vi "OPO Monitor.vi"() -> ()   [LabVIEW 2009]
doc: "Example: Simulated Acquisition\n\nRecommended Input Signal: None\n\nDevices Supported: NI 5102, NI 5911, NI 5112, NI 5620, NI 5621, NI 5122, NI 5124, NI 5922, NI 5114, NI 5142 (562x devices require configuration of a 2 V vertical range, 50 ohm input impedance and appropriate vertical coupling).\n\nDescription:\n\nThis example simulates an acquisition on the selected digitizer. To select a digitizer choose a model and a board type from the menu rings. Not all models support all board types. For example, there is only a PXI-5620, but there all the board types exist for a NI-5102.\n\nThis example configures all the digitizer's vertical, horizontal, and triggering properties before every acquisition. It allows you to experiment with numerous configurations, including some triggering modes, since it supports nearly the entire functionality of NI-SCOPE.\n\nMany parameters are included an the front panel of this example. Notice that the \"min sample rate\" is next to the \"actual sample rate,\" and similarly the \"min record length\" is near the \"actual record length.\" The \"min\" values are specified with the Configure Horizontal Timing VI. NI-SCOPE maintains a constant time per record for each acquisition. So when you specify a min sample rate and a min record length, this determines the amount of time the acquisition should take:\n\n time per record = min record length / min sampling rate. \n\nHowever, digitizers support only a certain number of defined sampling rates, so if the value chosen is not a valid rate, it is rounded to the next higher rate, called the actual sample rate. The actual record length is then calculated in order to maintain the time per record. Both of these values are returned in this example so you can investigate the effects of parameter rounding with your digitizer. For more information about parameter coercions, see the NI High Speed Digitizers Help.\n\nThe enforce realtime property allows this example to use Random Interleaved Sampling. See the Random Interleaved Sampling example for more details.\n\nKeep in mind that not all digitizers support all the features in this example. The NI High Speed Digitizers Help includes a table of supported features for each device."
uses:
  <instrlib>/niScope/Controls/niScope vertical coupling.ctl
  Pulse Acquisition/5122-States.ctl
  <instrlib>/niScope/Configure/Trigger/niScope Configure Trigger Edge.vi
  <instrlib>/niScope/Acquire/Fetch/niScope Fetch.vi
  <vilib>/Utility/file.llb/Write To Spreadsheet File (DBL).vi
panel:
  in  "Resource name 5":refnum<k15>="Dev2" caption="Resource Name"
  in  "Channel name (0 or 1) 6":string="0" caption="Channel Name(s)"
  in  "Vertical range (0 to 10V) 6":dbl=0.2 caption="Vertical Range (V)" format="%.2f"
  in  "Sample rate 6":dbl=100000000.0 caption="Min. Sample Rate" step=1000000.0 format="%.3p"
  in  "Number of points\n(max 23500000 si \n100 Ms/s) 5":i32=1000000 caption="Min. Record Length"
  in  "Trigger slope 6":i32(ring) caption="Trigger Slope" items=["Positive", "Negative"]
  in  "Trigger level 5":dbl=0.5 caption="Trigger Level" format="%.2f"
  in  "Trigger source 5":string(combo)="VAL_EXTERNAL" caption="Trigger Source"
  in  "Vertical coupling 6":T1 caption="Vertical Coupling" items=["AC", "DC", "Ground"]
  out "Acquisition time (s) 5":dbl
  in  "Delay trig to acquisition (s) 5":dbl=0.0001 format="%#_7e"
  in  "Capture":bool
  in  "Stop acquisition":bool
  in  "File where data is written":path=path "C:/Users/atomes/Documents/Manips/Labview manip/SQZ/Acquisition brute carte/Data acquisition.txt"
  out "Acquisition brute carte":dbl[](graph)
  # "General"
  # "Timing control"
  # "Trigger"
  # "Vertical"
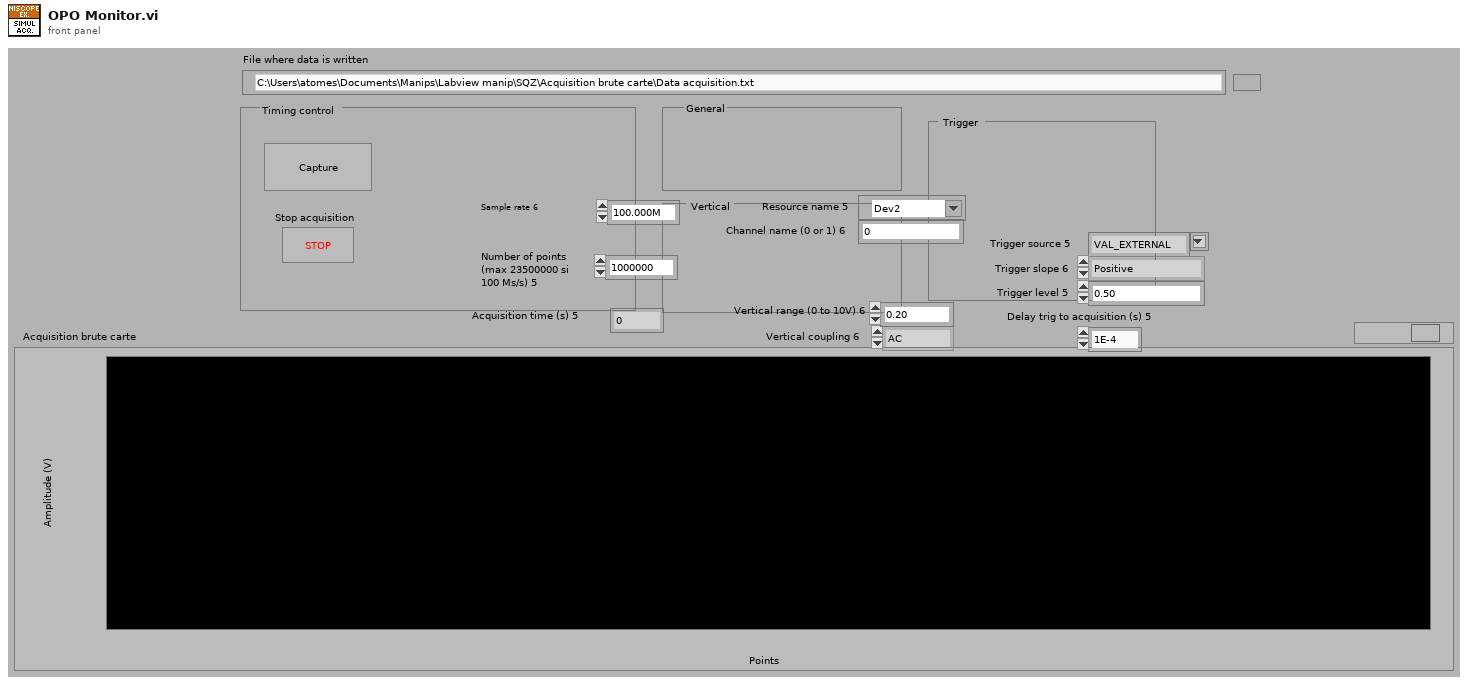
[diagram p1: front panel]
types:
  T1 = typedef "niScope vertical coupling.ctl" = i32
  T2 = typedef "5122-States.ctl" = enum16{"Initialize Card", "Continuous Mode", "Fetch", "Snapshot Acquistion", "Standby", "Record DataFile", "Exit"}
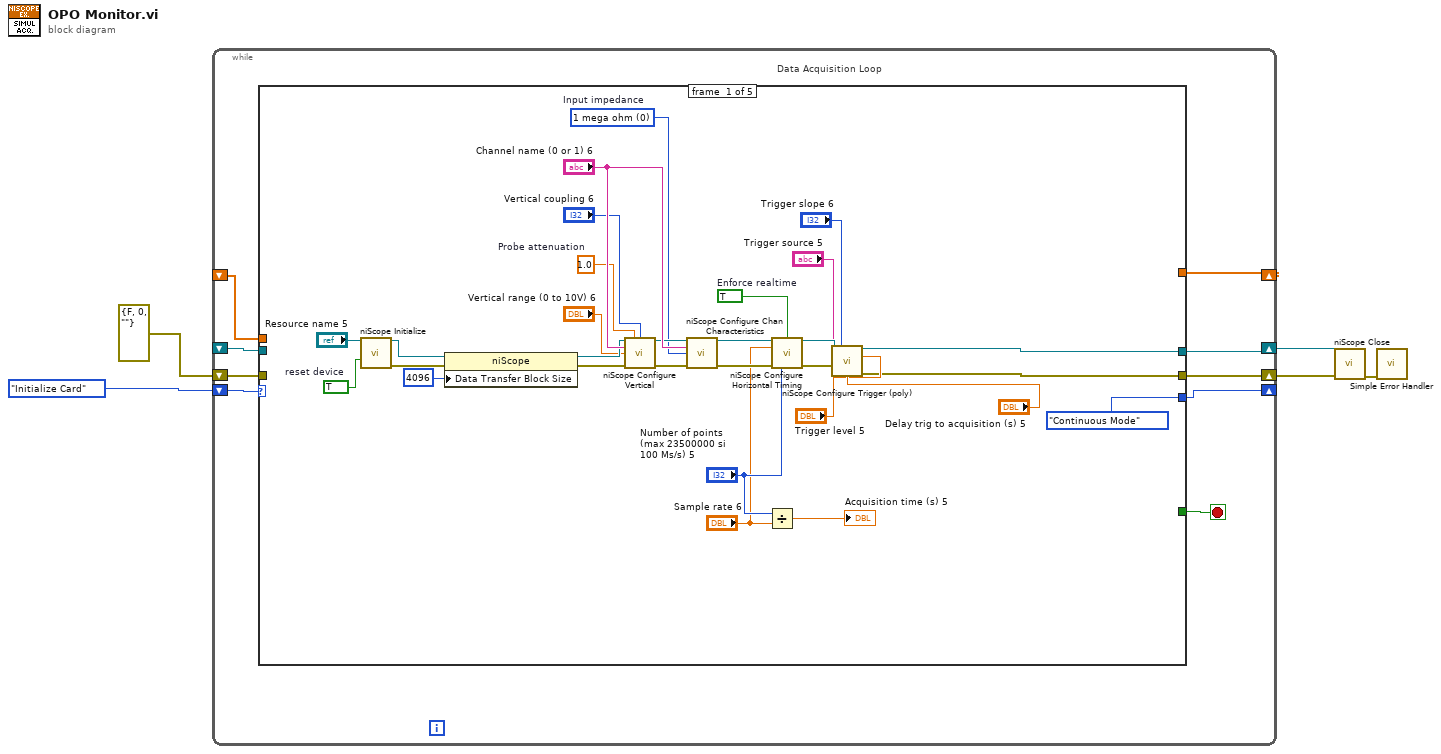
[diagram p0: block diagram]
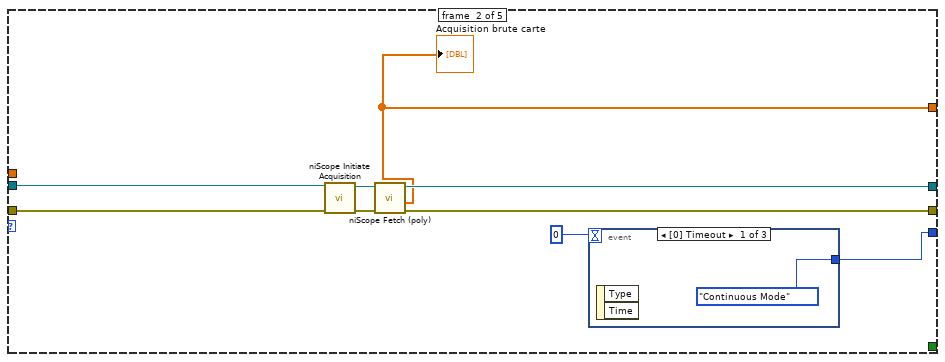
[diagram p2: hidden frame]
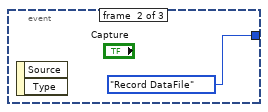
[diagram p3: hidden frame]
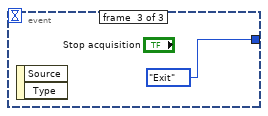
[diagram p4: hidden frame]
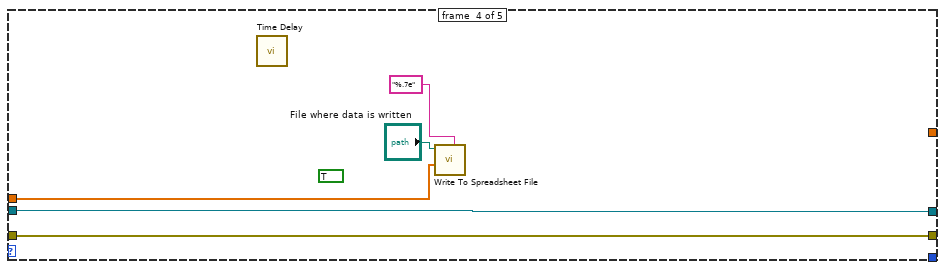
[diagram p6: hidden frame]
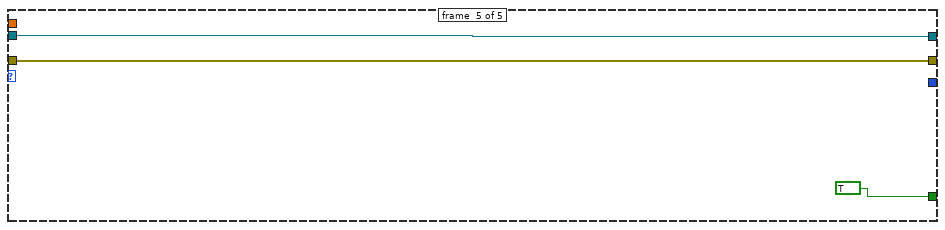
[diagram p7: hidden frame]
diagram:
  n1 = while {
    shift-right: [w9] -> _
    shift-left: 5122-States."Initialize Card" ("Enum") -> [w14]
    shift-right: [w13] -> w3
    shift-left: _ -> [w11]
    shift-right: [w12] -> w2
    shift-left: errorcluster {"status"=FALSE, "code"=0, "source"=""} ("error out") -> [w10]
    shift-right: [w7] -> _
    shift-left: _ -> [w6]
    stop <- w8 stop-if-true
    # "Data Acquisition Loop"
    n2 = case shown="\"Continuous Mode\"" w14 {
      tunnel: [w17 w46 w57 w62 w64] -> w13
      tunnel: [w16 w45 w56 w61 w63] -> w12
      tunnel: w11 -> [_ w52 w57 w62 w64]
      tunnel: w10 -> [_ w51 w56 w61 w63]
      tunnel: [5122-States."Continuous Mode" ("Enum") w47 _ _ _] -> w9
      tunnel: [_ _ _ _ TRUE] -> w8
      tunnel: [_ w44 _ _ _] -> w7
      tunnel: w6 -> [_ _ _ w58 _]
      frame #0 {
        w32 = TRUE  # Enforce realtime
        w18 = 1.0  # Probe attenuation
        w28 = u32 0 items=["1 mega ohm", "75 ohms", "50 ohms"]  # Input impedance
        w38 = TRUE  # reset device
        n3 = call <instrlib>:"niScope Initialize.vi"("resource name"="Resource name 5", "reset device"=w38) -> ("instrument handle"=w36:refnum<k15>, "error out"=w35:errorcluster)  [unwired: 2 in, 10 out]
        n4 = property class="niScope"(reference=w36, error in=w35, "Data Transfer Block Size"=4096) -> (reference out=w39:refnum<k15>, error out=w40:errorcluster)
        n5 = call <instrlib>:"niScope Configure Vertical.vi"("instrument handle"=w39, "probe attenuation"=w18, "vertical coupling"="Vertical coupling 6", "channels"="Channel name (0 or 1) 6", "vertical range"="Vertical range (0 to 10V) 6", "error in"=w40) -> ("instrument handle out"=w31:refnum<k15>, "error out"=w30:errorcluster)  [unwired: 2 in, 6 out]
        n6 = call <instrlib>:"niScope Configure Chan Characteristics.vi"("instrument handle"=w31, "channels"="Channel name (0 or 1) 6", "input impedance"=w28, "error in"=w30) -> ("instrument handle out"=w19:refnum<k15>, "error out"=w29:errorcluster)  [unwired: 1 in, 9 out]
        n7 = Divide(x="Number of points\n(max 23500000 si \n100 Ms/s) 5", y="Sample rate 6") -> (x/y=→"Acquisition time (s) 5":dbl)
        n8 = call <instrlib>:"niScope Configure Horizontal Timing.vi"("instrument handle"=w19, "enforce realtime"=w32, "min sample rate"="Sample rate 6", "error in"=w29, "min record length"="Number of points\n(max 23500000 si \n100 Ms/s) 5") -> ("instrument handle out"=w26:refnum<k15>, "error out"=w27:errorcluster)  [unwired: 2 in, 7 out]
        n9 = call-poly <instrlib>:"niScope Configure Trigger (poly).vi"("instrument handle"=w26, "trigger slope"="Trigger slope 6", "trigger source"="Trigger source 5", "trigger level"="Trigger level 5", "error in"=w27, "trigger delay"="Delay trig to acquisition (s) 5") -> ("instrument handle out"=w17:refnum<k15>, "error out"=w16:errorcluster)  [unwired: 2 in, 6 out]
      }
      frame #1 {
        n10 = call <instrlib>:"niScope Initiate Acquisition.vi"("instrument handle"=w52, "error in"=w51) -> ("instrument handle out"=w50:refnum<k15>, "error out"=w49:errorcluster)  [unwired: 12 out]
        n11 = call-poly <instrlib>:"niScope Fetch (poly).vi"("error in"=w49, "instrument handle"=w50) -> ("error out"=w45:errorcluster, "wfm"=w44:dbl[], "instrument handle out"=w46:refnum<k15>)  [unwired: 3 in, 4 out]
        "Acquisition brute carte" <- w44
        n12 = event shown="[0] Timeout" {
          selector: _ -> [_ _ _]
          dyn-events: _ -> [_ _ _]
          timeout: 0 -> [_ _ _]
          tunnel: [5122-States."Continuous Mode" ("Enum") 5122-States."Record DataFile" ("Enum") 5122-States."Exit" ("Enum")] -> w47
          event #0 {
            n13 = event-data() -> ()  [unwired: 3 out]
          }
          event #1 {
            n14 = event-data() -> ()  [unwired: 3 out]
          }
          event #2 {
            n15 = event-data() -> ()  [unwired: 3 out]
          }
        }
      }
      frame #2 {
      }
      frame #3 {
        (unwired) TRUE
        n16 = call "Time Delay"() -> ()  [unwired: 2 in, 10 out]
        n17 = call-poly <vilib>:"Write To Spreadsheet File.vi"("format (%.3f)"="%.7e", "1D data"=w58, "file path (dialog if empty)"="File where data is written") -> ()  [unwired: 3 in, 3 out]
      }
      frame #4 {
      }
    }
  }
  n18 = call <instrlib>:"niScope Close.vi"("instrument handle"=w3, "error in"=w2) -> ("error out"=w4:errorcluster)  [unwired: 13 out]
  n19 = call <vilib>:"Simple Error Handler.vi"("error in (no error)"=w4) -> ()  [unwired: 1 in, 8 out]
